vi "PushCameFrom.vi"(1 "CameFrom":T1, 2 "nó atual":cluster{"id":dbl, "x":dbl, "y":dbl}, 3 "nó pai":cluster{"id":dbl, "x":dbl, "y":dbl}) -> (9 "CameFromOut":cluster{"id":dbl, "x":dbl, "y":dbl}[][](array[cluster]))   [LabVIEW 2016]
uses:
  CameFrom.ctl
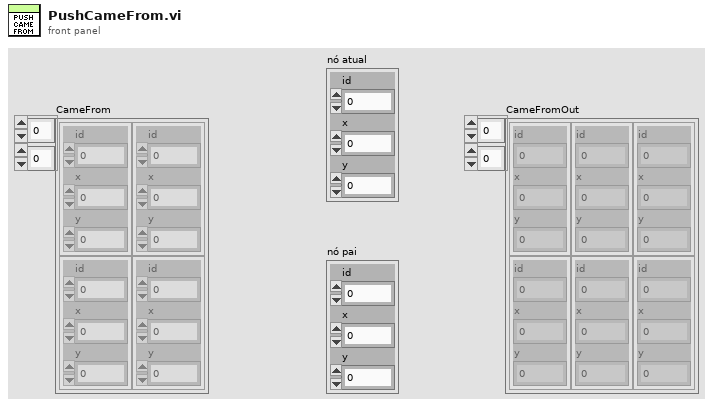
[diagram p1: front panel]
types:
  T1 = typedef "CameFrom.ctl" = cluster{"id":dbl, "x":dbl, "y":dbl}[][]
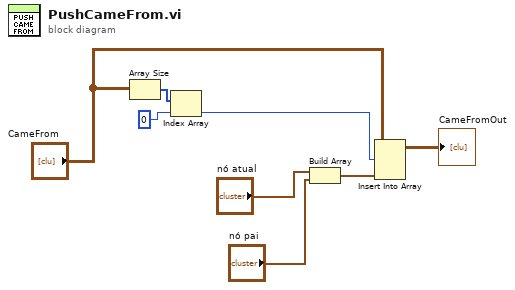
[diagram p0: block diagram]
diagram:
  n1 = Array Size(array="CameFrom") -> (size(s)=w8:i32[])
  n2 = Index Array(array=w8, index=0) -> (element=w6:i32)
  n3 = Build Array("nó atual", "nó pai") -> (w3:cluster{"id":dbl, "x":dbl, "y":dbl}[])
  n4 = Insert Into Array(array="CameFrom", index (row)=w6, new element=w3) -> (→"CameFromOut":T1)  [unwired: 1 in]
